vi "SMU Switch Handshaking - 1A - 2810 - Ba.vi"(8 "error in":errorcluster, 11 "file path (use dialog)":path=path "C:/Users/IES/Desktop/jsontestfile.json") -> (0 "error out":errorcluster, 1 "Ba Results":T1[](array[typedef]) {"Impedance" format="%#_6p"; "Negative Voltage" format="%#_6p"; "Positive Voltage" format="%#_6p"}, 2 "Results":T4={"R ch0 Array"=[2.6402355104591723e-06, 3.2050422226470716e-06, 3.2738385547093894e-06, 3.0004056082675545e-06, 3.190429018678622e-06, 3.265655292871135e-06, 3.4283206777974678e-06], "R ch1 Array"=[3.579181433209794e-06, 3.538102305000126e-06, 3.3674070559982216e-06, 3.2951997357567907e-06, 3.0614196043446336e-06, 3.247982674682344e-06, 3.4582756481500834e-06], "R ch2 Array"=[2.636942617106564e-06, 2.444215695573972e-06, 2.3600385872845126e-06, 2.3785120159418297e-06, 2.39158079459529e-06, 2.5415574149365358e-06, 2.629696833600491e-06], "R ch3 Array"=[4.29015971742814e-06, 4.582682915243894e-06, 4.199947801068903e-06, 4.210565880465411e-06, 4.1249236933492e-06, 4.3283146693326225e-06], "R ch4 Array"=[3.2068632920738282e-06, 3.2352868353418705e-06, 3.218523090660476e-06, 3.1985005992771743e-06, 3.2252632419667723e-06, 3.3472279144313767e-06], "R ch5 Array"=[4.190513905088153e-06, 4.23972086032935e-06, 4.053579560688339e-06, 3.9410571545407844e-06, 4.234836387112458e-06, 4.06030163753006e-06], "Elapsed Time (ms)"=11164, "SMU Fault Array"=[], "DMM Fault Array"=[]} {"R ch0 Array" format="%#_6p"; "R ch3 Array" format="%#_6p"; "R ch1 Array" format="%#_6p"; "R ch4 Array" format="%#_6p"; "R ch2 Array" format="%#_6p"; "R ch5 Array" format="%#_6p"}, 3 "Elapsed Time":u32)   [LabVIEW 2019]
uses:
  Results.ctl
  <instrlib>/niDMM/nidmm.llb/niDMM Acquisition State.ctl
  Labview-grpc-measurement-server-master/VIs/MeasurementServer_FourProbeRawData.ctl
  Labview-grpc-measurement-server-master/VIs/MeasurementServer_ErrorOutData.ctl
  JSONCluster.ctl
  <instrlib>/niDCPower/nidcpower.llb/niDCPower Send Software Edge Trigger - Signal.ctl
  <instrlib>/niSwitch/niSwitch.llb/niSwitch Topologies.ctl
  <instrlib>/niDMM/nidmm.llb/niDMM Configure Measurement Absolute.vi
  <instrlib>/niDCPower/nidcpower.llb/niDCPower Configure Software Edge Start Trigger.vi
  <instrlib>/niDCPower/nidcpower.llb/niDCPower Configure Software Edge Sequence Advance Trigger.vi
  <instrlib>/niSwitch/niSwitch.llb/niSwitch Connect Channels (Multiple).vi
  <instrlib>/niSwitch/niSwitch.llb/niSwitch Connect Channels (Single).vi
  <instrlib>/niSwitch/niSwitch.llb/niSwitch Disconnect Channels (Single).vi
  <instrlib>/niSwitch/niSwitch.llb/niSwitch Disconnect Channels (Multiple).vi
  Labview-grpc-measurement-server-master/VIs/labview-grpc-measurement-server.lvlib
panel:
  out "Acq State":T3 caption="Acquisition State"
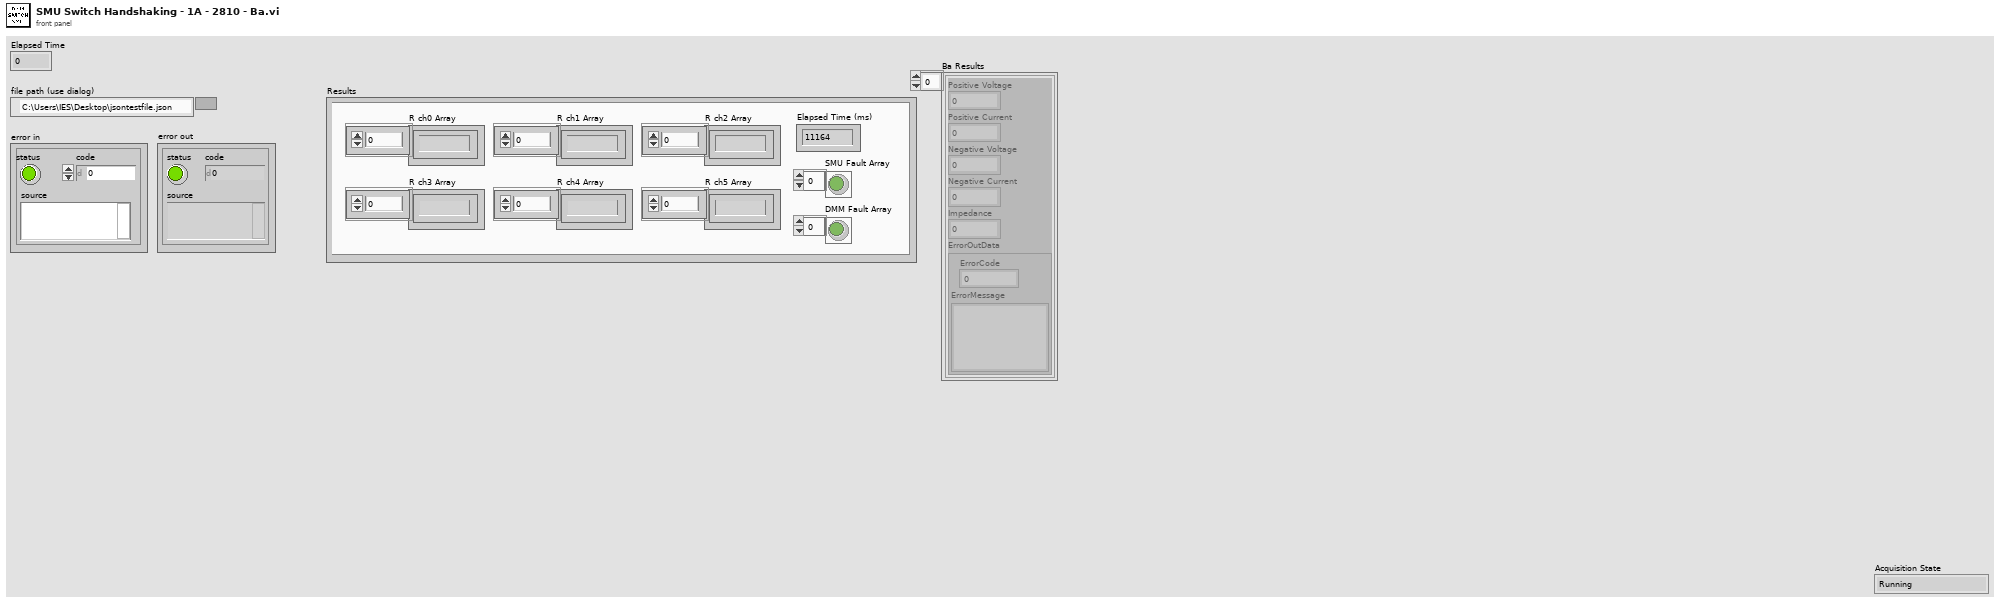
[diagram p1: front panel]
types:
  T1 = typedef "labview-grpc-measurement-server.lvlib/MeasurementServer_FourProbeRawData.ctl" = cluster{"Positive Voltage":sgl, "Positive Current":sgl, "Negative Voltage":sgl, "Negative Current":sgl, "Impedance":sgl, "ErrorOutData":T2}
  T2 = typedef "labview-grpc-measurement-server.lvlib/MeasurementServer_ErrorOutData.ctl" = cluster{"ErrorCode":i32, "ErrorMessage":string}
  T3 = typedef "niDMM Acquisition State.ctl" = enum16{"Running", "Finished with Backlog", "Finished with no Backlog", "Paused", "No acquisition in progress"}
  T4 = typedef "Results.ctl" = cluster{"R ch0 Array":dbl[], "R ch1 Array":dbl[], "R ch2 Array":dbl[], "R ch3 Array":dbl[], "R ch4 Array":dbl[], "R ch5 Array":dbl[], "Elapsed Time (ms)":u32, "SMU Fault Array":bool[], "DMM Fault Array":bool[]}
  T5 = typedef "niSwitch Topologies.ctl" = string
  T6 = typedef "niDCPower Send Software Edge Trigger - Signal.ctl" = i32
  T7 = typedef "JSONCluster.ctl" = cluster{"SMUResourceName":string, "SMUChannels":string, "SMUSourceMode_Sequence":i32, "SMUOutputFunction_DCCurrent":i32, "SMUSourceTransientResponse_Fast":i32, "SMUCurrent":dbl, "SMUCurrentLevelRange":dbl, "SMUMeasurementSense_Local":i32, "SMUMeasurementApertureTime":dbl, "SMUSourceAdvancedSourceDelay":dbl, "SMUVoltage":dbl, "SMUSourceAdvancedSequenceLoopCount":i32, "SMUMeasurementAdvancedDCNoiseRejection_Normal":i32, "SMUSequenceName":string, "SMUStep1_Source_DCCurrent_CurrentLevel":i32, "SMUStep2_Measurement_ApertureTime":i32, "SMUStep3_Source_Advanced_SourceDelay":i32, "SMUSequenceNumberOfSteps":i32, "SMUTriggerFromSwitch_StartDigitalEdge":string, "SMUTriggerFromSwitch_SequenceAdvanceDigitalEdge":string, "SMUTriggerToDMM_SourceCompleteEvent":i32, "SMUTriggerToDMM_SourceCompleteEvent_Value":string, "SMUTriggerToSwitch_SequenceIterationCompleteEvent":i32, "SMUTriggerToDMM_SequenceIterationCompleteEvent_Value":string, "SwitchResourceName":string, "SwitchTopology":string, "SwitchInputTrigger_TTL0":i32, "SwitchScanAdvancedOutput_TTL1":i32, "SwitchScanList":string, "DMMResourceName":string, "DMMFunction_DCVolts":i32, "DMMResolution":dbl, "DMMRange":dbl, "DMMTriggerSource_TTL2":i32, "DMMTriggerSlope_RisingEdge":i32, "DMMSampleTrigger_TTL2":i32, "DMMSampleCount":i32, "DMMSampleTriggerSlope_RisingEdge":i32, "DMMApertureTimeUnits_Seconds":i32, "DMMApertureTime":dbl, "DMMNumberOfAverages":i32, "DMMAutoZero_Off":i32, "DMMADCCalibration_Off":i32, "DMMSettleTime":dbl, "DMMControlAction_Commit":i32, "ApplicationNumberOfWeldChannels":i32}
  T8 = enum16{"open", "replace", "create", "open or create", "replace or create", "replace or create with confirmation"}
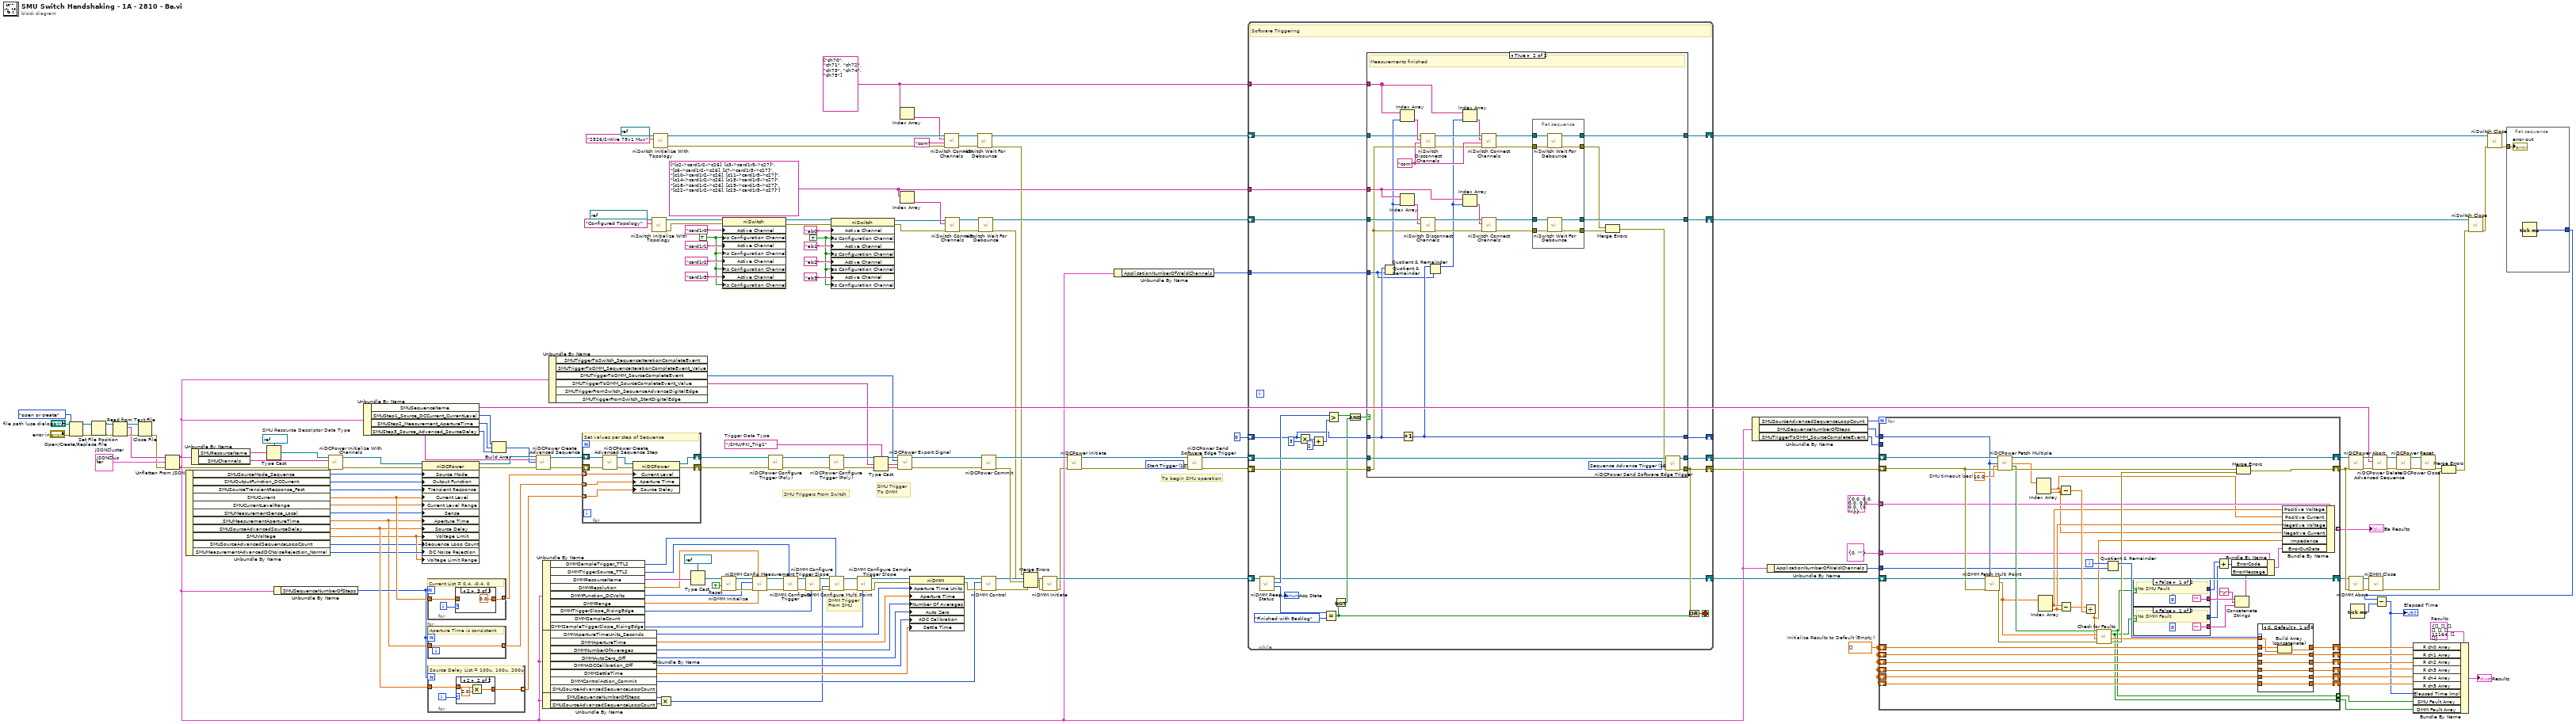
[diagram p0: block diagram]
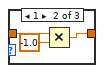
[diagram p4: hidden frame]
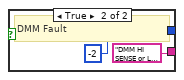
[diagram p6: hidden frame]
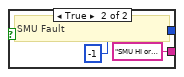
[diagram p7: hidden frame]
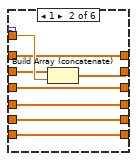
[diagram p8: hidden frame]
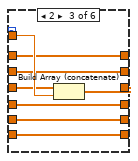
[diagram p9: hidden frame]
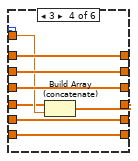
[diagram p10: hidden frame]
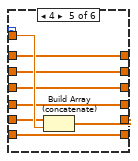
[diagram p11: hidden frame]
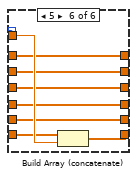
[diagram p12: hidden frame]
diagram:
  w10 = string[] ["ch70", "ch71", "ch72", "ch73", "ch74", "ch75"] ("2525 Scan List Channels")
  w22 = TRUE ("Channel Configuration:Analog Bus Sharing Enable")
  w35 = string[] ["[c2->card1r2->c26], [c3->card1r3->c27]", "[c6->card1r2->c26], [c7->card1r3->c27]", "[c10->card1r2->c26], [c11->card1r3->c27]", "[c14->card1r2->c26], [c15->card1r3->c27]", "[c18->card1r2->c26], [c19->card1r3->c27]", "[c22->card1r2->c26], [c23->card1r3->c27]"]
  w36 = TRUE ("Channel Configuration:Is Source Channel")
  w57 = T6 1034 items=["Start Trigger"=1034, "Source Trigger"=1035, "Measure Trigger"=1036, "Sequence Advance Trigger"=1037, "Pulse Trigger"=1053] ("signal")
  w134 = refnum<k15> "SMU"  # SMU Resource Descriptor Data Type
  w130 = T7 {"SMUResourceName"="", "SMUChannels"="", "SMUSourceMode_Sequence"=0, "SMUOutputFunction_DCCurrent"=0, "SMUSourceTransientResponse_Fast"=0, "SMUCurrent"=0.0, "SMUCurrentLevelRange"=0.0, "SMUMeasurementSense_Local"=0, "SMUMeasurementApertureTime"=0.0, "SMUSourceAdvancedSourceDelay"=0.0, "SMUVoltage"=0.0, "SMUSourceAdvancedSequenceLoopCount"=0, "SMUMeasurementAdvancedDCNoiseRejection_Normal"=0, "SMUSequenceName"="", "SMUStep1_Source_DCCurrent_CurrentLevel"=0, "SMUStep2_Measurement_ApertureTime"=0, "SMUStep3_Source_Advanced_SourceDelay"=0, "SMUSequenceNumberOfSteps"=0, "SMUTriggerFromSwitch_StartDigitalEdge"="", "SMUTriggerFromSwitch_SequenceAdvanceDigitalEdge"="", "SMUTriggerToDMM_SourceCompleteEvent"=0, "SMUTriggerToDMM_SourceCompleteEvent_Value"="", "SMUTriggerToSwitch_SequenceIterationCompleteEvent"=0, "SMUTriggerToDMM_SequenceIterationCompleteEvent_Value"="", "SwitchResourceName"="", "SwitchTopology"="", "SwitchInputTrigger_TTL0"=0, "SwitchScanAdvancedOutput_TTL1"=0, "SwitchScanList"="", "DMMResourceName"="", "DMMFunction_DCVolts"=0, "DMMResolution"=0.0, "DMMRange"=0.0, "DMMTriggerSource_TTL2"=0, "DMMTriggerSlope_RisingEdge"=0, "DMMSampleTrigger_TTL2"=0, "DMMSampleCount"=0, "DMMSampleTriggerSlope_RisingEdge"=0, "DMMApertureTimeUnits_Seconds"=0, "DMMApertureTime"=0.0, "DMMNumberOfAverages"=0, "DMMAutoZero_Off"=0, "DMMADCCalibration_Off"=0, "DMMSettleTime"=0.0, "DMMControlAction_Commit"=0, "ApplicationNumberOfWeldChannels"=0}  # JSONCluster
  w115 = T4 {"R ch0 Array"=[], "R ch1 Array"=[], "R ch2 Array"=[], "R ch3 Array"=[], "R ch4 Array"=[], "R ch5 Array"=[], "Elapsed Time (ms)"=11164, "SMU Fault Array"=[], "DMM Fault Array"=[]}  # Results
  w117 = dbl[] []  # Initialize Results to Default (Empty)
  w162 = TRUE  # Reset
  w84 = tag "/SMU/PXI_Trig1"  # Trigger Data Type
  # "To begin SMU operation"
  # "DMM Trigger\nFrom SMU"
  # "SMU Trigger \nTo DMM"
  # "SMU Triggers From Switch"
  n1 = Open/Create/Replace File(file path (use dialog)="file path (use dialog)", error in="error in", operation (0:open)=T8."open or create") -> (refnum out=w123:refnum<file>, error out=w122:errorcluster)  [unwired: 3 in, 1 out]
  n2 = Set File Position(refnum=w123, error in=w122) -> (refnum out=w125:refnum<file>, error out=w124:errorcluster)  [unwired: 2 in]
  n3 = Read from Text File(file (use dialog)=w125, error in=w124) -> (refnum out=w127:refnum<file>, text=w121:string, error out=w126:errorcluster)  [unwired: 2 in, 1 out]
  n4 = Close File(refnum=w127, error in=w126) -> (error out=w120:errorcluster)  [unwired: 1 out]
  n5 = Unflatten From JSON(JSON string=w121, type and defaults=w130, error in (no error)=w120) -> (value=w47:T7, error out=w119:errorcluster)  [unwired: 4 in]
  n6 = Unbundle By Name(w47) -> ("SMUSourceMode_Sequence"=w97:i32, "SMUOutputFunction_DCCurrent"=w96:i32, "SMUSourceTransientResponse_Fast"=w102:i32, "SMUCurrent"=w101:dbl, "SMUCurrentLevelRange"=w100:dbl, "SMUMeasurementSense_Local"=w99:i32, "SMUMeasurementApertureTime"=w6:dbl, "SMUSourceAdvancedSourceDelay"=w98:dbl, "SMUVoltage"=w94:dbl, "SMUSourceAdvancedSequenceLoopCount"=w69:i32, "SMUMeasurementAdvancedDCNoiseRejection_Normal"=w95:i32)
  n7 = Unbundle By Name(w47) -> ("SMUResourceName"=w132:string, "SMUChannels"=w131:string)
  n8 = Type Cast(type=w134, x=w132) -> (*(type *) &x=w133:refnum<k15>)
  n9 = Unbundle By Name(w47) -> ("SMUSequenceNumberOfSteps"=w92:i32)
  n10 = call <instrlib>:"niDCPower Initialize With Channels.vi"("error in (no error)"=w119, "channels"=w131, "resource name"=w133) -> ("error out"=w181:errorcluster, "instrument handle out"=w182:refnum<k15>)  [unwired: 7 in]
  n11 = Unbundle By Name(w47) -> ("SMUSequenceName"=w88:string, "SMUStep1_Source_DCCurrent_CurrentLevel"=w91:i32, "SMUStep2_Measurement_ApertureTime"=w90:i32, "SMUStep3_Source_Advanced_SourceDelay"=w89:i32)
  n12 = property class="niDCPower"(reference=w182, error in=w181, "Source Mode"=w97, "Output Function"=w96, "Transient Response"=w102, "Current Level"=w101, "Current Level Range"=w100, "Sense"=w99, "Aperture Time"=w6, "Source Delay"=w98, "Voltage Limit"=w94, "Sequence Loop Count"=w69, "DC Noise Rejection"=w95, "Voltage Limit Range"=w94) -> (reference out=w176:refnum<k15>, error out=w175:errorcluster)
  n13 = for {
    N: w92 -> [_]
    tunnel: w101 -> [w184]
    tunnel: [w183] -> w105 mode=indexing
    i -> [w185]
    # "Current List = 0.4, -0.4, 0"
    n14 = case shown="2" w185 {
      tunnel: w184 -> [w186 w188 _]
      tunnel: [w186 w189 0.0 ("current")] -> w183
      frame 0, Default {
      }
      frame 1 {
        n15 = Multiply(x=w188, y=-1.0) -> (x*y=w189:dbl)
      }
      frame 2 {
      }
    }
  }
  n16 = for {
    N: w92 -> [_]
    tunnel: w6 -> [w191]
    tunnel: [w191] -> w104 mode=indexing
    # "Aperture Time is consistent"
  }
  n17 = for {
    N: w92 -> [_]
    tunnel: w98 -> [w194]
    tunnel: [w193] -> w103 mode=indexing
    i -> [w192]
    # "Source Delay List = 100u, 100u, 200u"
    n18 = case shown="2" w192 {
      tunnel: w194 -> [w195 w198]
      tunnel: [w195 w196] -> w193
      frame 0, Default {
      }
      frame 2 {
        n19 = Multiply(x=w198, y=2.0) -> (x*y=w196:dbl)
      }
    }
  }
  n20 = Build Array(w91, w90, w89) -> (w93:i32[])
  n21 = call <instrlib>:"niDCPower Create Advanced Sequence.vi"("instrument handle"=w176, "sequence name"=w88, "advanced sequence properties"=w93, "error in (no error)"=w175) -> ("instrument handle out"=w168:refnum<k15>, "error out"=w167:errorcluster)  [unwired: 10 in]
  n22 = Unbundle By Name(w47) -> ("DMMSampleTrigger_TTL2"=w76:i32, "DMMTriggerSource_TTL2"=w81:i32, "DMMResourceName"=w64:string, "DMMResolution"=w63:dbl, "DMMFunction_DCVolts"=w78:i32, "DMMRange"=w80:dbl, "DMMTriggerSlope_RisingEdge"=w79:i32, "DMMSampleTriggerSlope_RisingEdge"=w77:i32)  [unwired: 1 out]
  n23 = Unbundle By Name(w47) -> ("DMMApertureTimeUnits_Seconds"=w75:i32, "DMMApertureTime"=w5:dbl, "DMMNumberOfAverages"=w74:i32, "DMMAutoZero_Off"=w73:i32, "DMMADCCalibration_Off"=w72:i32, "DMMSettleTime"=w71:dbl, "DMMControlAction_Commit"=w70:i32)  [unwired: 1 out]
  n24 = Unbundle By Name(w47) -> ("SMUSequenceNumberOfSteps"=w53:i32, "SMUSourceAdvancedSequenceLoopCount"=w52:i32)
  n25 = Unbundle By Name(w47) -> ("SMUTriggerToDMM_SourceCompleteEvent"=w87:i32, "SMUTriggerToDMM_SourceCompleteEvent_Value"=w85:string)  [unwired: 4 out]
  n26 = for {
    shift-right: [w204] -> w165
    shift-left: w167 -> [w207]
    shift-right: [w203] -> w166
    shift-left: w168 -> [w202]
    tunnel: w103 -> [w201] mode=indexing
    tunnel: w105 -> [w199] mode=indexing
    tunnel: w104 -> [w200] mode=indexing
    # "Set values per step of Sequence"
    n27 = call <instrlib>:"niDCPower Create Advanced Sequence Step.vi"("error in (no error)"=w207, "instrument handle"=w202) -> ("error out"=w205:errorcluster, "instrument handle out"=w206:refnum<k15>)  [unwired: 8 in]
    n28 = property class="niDCPower"(reference=w206, error in=w205, "Current Level"=w199, "Aperture Time"=w200, "Source Delay"=w201) -> (reference out=w203:refnum<k15>, error out=w204:errorcluster)
  }
  n29 = call <instrlib>:"niSwitch Initialize With Topology.vi"("topology name"=T5 "Configured Topology", "resource name"=refnum<k15> "SwitchBlock1Dev1") -> ("error out"=w41:errorcluster, "instrument handle out"=w42:refnum<k15>)  [unwired: 3 in, 5 out]
  n30 = call <instrlib>:"niSwitch Initialize With Topology.vi"("topology name"=T5 "2526/2-Wire 79x1 Mux", "resource name"=refnum<k15> "2526_1") -> ("error out"=w18:errorcluster, "instrument handle out"=w19:refnum<k15>)  [unwired: 3 in, 5 out]
  n31 = Multiply(x=w53, y=w52) -> (x*y=w51:i32)
  n32 = Type Cast(type=refnum<k15> "DMM" ("Device Name"), x=w64) -> (*(type *) &x=w82:refnum<k15>)
  n33 = call <instrlib>:"niDMM Initialize.vi"("Reset"=w162, "Instrument Descriptor"=w82) -> ("error out"=w151:errorcluster, "instrument handle out"=w150:refnum<k15>)  [unwired: 8 in]
  n34 = property class="niSwitch"(reference=w42, error in=w41, "Active Channel"="card1r0", "Is Configuration Channel"=w36, "Active Channel"="card1r1", "Is Configuration Channel"=w36, "Active Channel"="card1r2", "Is Configuration Channel"=w36, "Active Channel"="card1r3", "Is Configuration Channel"=w36) -> (reference out=w30:refnum<k15>, error out=w29:errorcluster)
  n35 = call-poly <instrlib>:"niDMM Config Measurement.vi"("Range"=w80, "Resolution"=w63, "error in (no error)"=w151, "Function"=w78, "instrument handle"=w150) -> ("error out"=w155:errorcluster, "instrument handle out"=w154:refnum<k15>)  [unwired: 5 in]
  n36 = call-poly <instrlib>:"niDCPower Configure Trigger (Poly).vi"("error in (no error)"=w165, "instrument handle"=w166) -> ("error out"=w178:errorcluster, "instrument handle out"=w179:refnum<k15>)  [unwired: 8 in]
  n37 = call <instrlib>:"niDMM Configure Trigger.vi"("Trigger Source"=w81, "error in (no error)"=w155, "instrument handle"=w154) -> ("error out"=w157:errorcluster, "instrument handle out"=w156:refnum<k15>)  [unwired: 7 in]
  n38 = call <instrlib>:"niDMM Configure Trigger Slope.vi"("Slope"=w79, "error in (no error)"=w157, "instrument handle"=w156) -> ("error out"=w159:errorcluster, "instrument handle out"=w158:refnum<k15>)  [unwired: 7 in]
  n39 = call-poly <instrlib>:"niDCPower Configure Trigger (Poly).vi"("error in (no error)"=w178, "instrument handle"=w179) -> ("error out"=w135:errorcluster, "instrument handle out"=w136:refnum<k15>)  [unwired: 8 in]
  n40 = call <instrlib>:"niDMM Configure Multi Point.vi"("Sample Trigger"=w76, "error in (no error)"=w159, "Sample Count"=w51, "instrument handle"=w158) -> ("error out"=w161:errorcluster, "instrument handle out"=w160:refnum<k15>)  [unwired: 6 in]
  n41 = property class="niSwitch"(reference=w30, error in=w29, "Active Channel"="ab0", "Is Configuration Channel"=w22, "Active Channel"="ab1", "Is Configuration Channel"=w22, "Active Channel"="ab2", "Is Configuration Channel"=w22, "Active Channel"="ab3", "Is Configuration Channel"=w22) -> (reference out=w28:refnum<k15>, error out=w27:errorcluster)
  n42 = call <instrlib>:"niDMM Configure Sample Trigger Slope.vi"("Slope"=w77, "error in (no error)"=w161, "instrument handle"=w160) -> ("error out"=w143:errorcluster, "instrument handle out"=w144:refnum<k15>)  [unwired: 7 in]
  n43 = Type Cast(type=w84, x=w85) -> (*(type *) &x=w86:tag)
  n44 = call <instrlib>:"niDCPower Export Signal.vi"("error in (no error)"=w135, "output terminal"=w86, "signal"=w87, "instrument handle"=w136) -> ("error out"=w163:errorcluster, "instrument handle out"=w164:refnum<k15>)  [unwired: 6 in]
  n45 = Index Array(array=w10) -> (element=w17:string)  [unwired: 1 in]
  n46 = Index Array(array=w35) -> (element=w48:string)  [unwired: 1 in]
  n47 = property class="niDMM"(reference=w144, error in=w143, "Aperture Time Units"=w75, "Aperture Time"=w5, "Number Of Averages"=w74, "Auto Zero"=w73, "ADC Calibration"=w72, "Settle Time"=w71) -> (reference out=w138:refnum<k15>, error out=w137:errorcluster)
  n48 = call-poly <instrlib>:"niSwitch Connect Channels.vi"("error in (no error)"=w18, "channel 2"="com", "channel 1"=w17, "instrument handle"=w19) -> ("error out"=w14:errorcluster, "instrument handle out"=w15:refnum<k15>)  [unwired: 6 in]
  n49 = call-poly <instrlib>:"niSwitch Connect Channels.vi"("error in (no error)"=w27, "connection list"=w48, "instrument handle"=w28) -> ("error out"=w33:errorcluster, "instrument handle out"=w34:refnum<k15>)  [unwired: 7 in]
  n50 = call <instrlib>:"niSwitch Wait For Debounce.vi"("error in (no error)"=w14, "instrument handle"=w15) -> ("error out"=w12:errorcluster, "instrument handle out"=w11:refnum<k15>)  [unwired: 8 in]
  n51 = call <instrlib>:"niSwitch Wait For Debounce.vi"("error in (no error)"=w33, "instrument handle"=w34) -> ("error out"=w32:errorcluster, "instrument handle out"=w31:refnum<k15>)  [unwired: 8 in]
  n52 = call <instrlib>:"niDCPower Commit.vi"("error in (no error)"=w163, "instrument handle"=w164) -> ("error out"=w149:errorcluster, "instrument handle out"=w146:refnum<k15>)  [unwired: 8 in]
  n53 = call <instrlib>:"niDMM Control.vi"("error in (no error)"=w137, "Control Action"=w70, "instrument handle"=w138) -> ("error out"=w148:errorcluster, "instrument handle out"=w145:refnum<k15>)  [unwired: 7 in]
  n54 = Merge Errors(w12, w32, w149, w148) -> (w147:errorcluster)
  n55 = call <instrlib>:"niDMM Initiate.vi"("error in (no error)"=w147, "instrument handle"=w145) -> ("error out"=w13:errorcluster, "instrument handle out"=w56:refnum<k15>)  [unwired: 8 in]
  n56 = call <instrlib>:"niDCPower Initiate.vi"("error in (no error)"=w13, "instrument handle"=w146) -> ("error out"=w45:errorcluster, "instrument handle out"=w60:refnum<k15>)  [unwired: 8 in]
  n57 = Unbundle By Name(w47) -> ("ApplicationNumberOfWeldChannels"=w46:i32)
  n58 = call <instrlib>:"niDCPower Send Software Edge Trigger.vi"("error in (no error)"=w45, "signal"=w57, "instrument handle"=w60) -> ("error out"=w58:errorcluster, "instrument handle out"=w59:refnum<k15>)  [unwired: 7 in]
  n59 = while {
    shift-right: [w234] -> w62
    shift-left: w59 -> [w229]
    shift-right: [w232] -> w61
    shift-left: w58 -> [w228]
    shift-right: [w230] -> w49
    shift-left: w31 -> [w231]
    shift-right: [w223] -> w55
    shift-left: w56 -> [w224]
    shift-right: [w217] -> _
    shift-left: 0 ("Backlog") -> [w218]
    tunnel: w35 -> [w212]
    tunnel: w46 -> [w211]
    shift-right: [w209] -> w9
    shift-left: w11 -> [w210]
    tunnel: w10 -> [w208]
    stop <- w233 stop-if-true
    # "Software Triggering"
    n60 = call <instrlib>:"niDMM Read Status.vi"("instrument handle"=w224) -> ("Acquisition State"=w227:T3, "Backlog"=w225:i32, "instrument handle out"=w223:refnum<k15>)  [unwired: 7 in, 1 out]
    "Acq State" <- w227
    n61 = Multiply(x=w218, y=3) -> (x*y=w220:i32)
    n62 = Add(x=w220, y=2) -> (x+y=w221:i32)
    n63 = Equal?(x=w227, y=niDMM_Acquisition_State."Finished with Backlog") -> (x = y?=w216:bool)
    n64 = Greater?(x=w225, y=w221) -> (0:w215:bool)
    n65 = Not(x=w216) -> (.not. x?=w214:bool)
    n66 = And(x=w215, y=w214) -> (x .and. y?=w213:bool)
    n67 = case shown="True" w213 {
      tunnel: w228 -> [w238 w243]
      tunnel: [w239 w271] -> w234
      tunnel: [w238 w270] -> w232
      tunnel: w229 -> [w239 w267]
      tunnel: w231 -> [w237 w266]
      tunnel: [w237 w269] -> w230
      tunnel: w218 -> [w236 w259]
      tunnel: [w236 w258] -> w217
      tunnel: w212 -> [_ w262]
      tunnel: w211 -> [_ w257]
      tunnel: w210 -> [w235 w248]
      tunnel: [w235 w245] -> w209
      tunnel: w208 -> [_ w244]
      frame False {
        # "Measurements not finished yet - repeat loop"
      }
      frame True {
        w252 = "com" ("channel 2")
        w268 = T6 1037 items=["Start Trigger"=1034, "Source Trigger"=1035, "Measure Trigger"=1036, "Sequence Advance Trigger"=1037, "Pulse Trigger"=1053] ("signal")
        # "Measurements finished"
        n68 = Quotient & Remainder(x=w259, y=w257) -> (x-y*floor(x/y)=w250:i32)  [unwired: 1 out]
        n69 = Index Array(array=w244, index=w250) -> (element=w255:string)
        n70 = Index Array(array=w262, index=w250) -> (element=w265:string)
        n71 = Increment(x=w259) -> (x+1=w258:i32)
        n72 = call-poly <instrlib>:"niSwitch Disconnect Channels.vi"("error in (no error)"=w243, "channel 2"=w252, "channel 1"=w255, "instrument handle"=w248) -> ("error out"=w251:errorcluster, "instrument handle out"=w254:refnum<k15>)  [unwired: 6 in]
        n73 = call-poly <instrlib>:"niSwitch Disconnect Channels.vi"("error in (no error)"=w243, "disconnection list"=w265, "instrument handle"=w266) -> ("error out"=w260:errorcluster, "instrument handle out"=w264:refnum<k15>)  [unwired: 7 in]
        n74 = Quotient & Remainder(x=w258, y=w257) -> (x-y*floor(x/y)=w249:i32)  [unwired: 1 out]
        n75 = Index Array(array=w244, index=w249) -> (element=w253:string)
        n76 = Index Array(array=w262, index=w249) -> (element=w261:string)
        n77 = call-poly <instrlib>:"niSwitch Connect Channels.vi"("error in (no error)"=w251, "channel 2"=w252, "channel 1"=w253, "instrument handle"=w254) -> ("error out"=w246:errorcluster, "instrument handle out"=w247:refnum<k15>)  [unwired: 6 in]
        n78 = call-poly <instrlib>:"niSwitch Connect Channels.vi"("error in (no error)"=w260, "connection list"=w261, "instrument handle"=w264) -> ("error out"=w256:errorcluster, "instrument handle out"=w263:refnum<k15>)  [unwired: 7 in]
        n79 = flat-sequence {
          tunnel: [w279] -> w269
          tunnel: [w278] -> w242
          tunnel: w263 -> [w277]
          tunnel: w256 -> [w276]
          tunnel: w247 -> [w275]
          tunnel: w246 -> [w274]
          tunnel: [w273] -> w245
          tunnel: [w272] -> w241
          frame #0 {
            n80 = call <instrlib>:"niSwitch Wait For Debounce.vi"("error in (no error)"=w274, "instrument handle"=w275) -> ("error out"=w272:errorcluster, "instrument handle out"=w273:refnum<k15>)  [unwired: 8 in]
            n81 = call <instrlib>:"niSwitch Wait For Debounce.vi"("error in (no error)"=w276, "instrument handle"=w277) -> ("error out"=w278:errorcluster, "instrument handle out"=w279:refnum<k15>)  [unwired: 8 in]
          }
        }
        n82 = Merge Errors(w241, w242) -> (w240:errorcluster)
        n83 = call <instrlib>:"niDCPower Send Software Edge Trigger.vi"("error in (no error)"=w240, "signal"=w268, "instrument handle"=w267) -> ("error out"=w270:errorcluster, "instrument handle out"=w271:refnum<k15>)  [unwired: 7 in]
      }
    }
    n84 = Or(x=w232, y=w216) -> (x .or. y?=w233:bool)
  }
  n85 = Unbundle By Name(w47) -> ("SMUSourceAdvancedSequenceLoopCount"=w68:i32, "SMUSequenceNumberOfSteps"=w67:i32, "SMUTriggerToDMM_SourceCompleteEvent"=w66:i32)
  n86 = Unbundle By Name(w47) -> ("ApplicationNumberOfWeldChannels"=w65:i32)
  n87 = for {
    N: w68 -> [_]
    tunnel: w67 -> [w302]
    shift-right: [w324] -> w142
    shift-left: w61 -> [w303]
    shift-right: [w329] -> w180
    shift-left: w62 -> [w304]
    shift-right: [w292] -> w139
    shift-left: w55 -> [w326]
    shift-right: [w323] -> w116
    shift-left: w117 -> [w322]
    shift-right: [w321] -> w110
    shift-left: w117 -> [w320]
    shift-right: [w319] -> w111
    shift-left: w117 -> [w318]
    shift-right: [w317] -> w112
    shift-left: w117 -> [w316]
    shift-right: [w315] -> w113
    shift-left: w117 -> [w314]
    shift-right: [w313] -> w114
    shift-left: w117 -> [w312]
    tunnel: [w287] -> w107 mode=indexing
    tunnel: [w283] -> w106 mode=indexing
    tunnel: w66 -> [_]
    tunnel: w65 -> [w301]
    tunnel: T1 {"Positive Voltage"=0.0, "Positive Current"=0.0, "Negative Voltage"=0.0, "Negative Current"=0.0, "Impedance"=0.0, "ErrorOutData"={"ErrorCode"=0, "ErrorMessage"=""}} ("FourProbeRawData") -> [w298]
    tunnel: T2 {"ErrorCode"=0, "ErrorMessage"=""} ("ErrorOutData") -> [w290]
    tunnel: [w289] -> w2 mode=indexing
    i -> [w328]
    w307 = 10.0  # SMU timeout (sec)
    n88 = call <instrlib>:"niDMM Fetch Multi Point.vi"("Number to Fetch"=w302, "error in (no error)"=w303, "instrument handle"=w326) -> ("error out"=w310:errorcluster, "Measurements"=w299:dbl[], "instrument handle out"=w292:refnum<k15>)  [unwired: 5 in, 1 out]
    n89 = call <instrlib>:"niDCPower Fetch Multiple.vi"("instrument handle"=w304, "count (1)"=w302, "timeout (sec)"=w307, "error in (no error)"=w303) -> ("instrument handle out"=w329:refnum<k15>, "current measurements"=w300:dbl[], "in compliance"=w311:bool[], "error out"=w325:errorcluster)  [unwired: 6 in, 2 out]
    n90 = Index Array(array=w300) -> (element #1=w296:dbl, element #2=w294:dbl)  [unwired: 2 in]
    n91 = Index Array(array=w299) -> (element #1=w297:dbl, element #2=w295:dbl)  [unwired: 2 in]
    n92 = Subtract(x=w296, y=w294) -> (x-y=w306:dbl)
    n93 = Subtract(x=w297, y=w295) -> (x-y=w305:dbl)
    n94 = Divide(x=w305, y=w306) -> (x/y=w293:dbl)
    n95 = call "Check for Faults.vi"("Error In"=w310, "Resistance In"=w293, "dmm voltage measurements"=w299, "in compliance"=w311) -> ("Error Out"=w309:errorcluster, "Resistance Out"=w308:dbl, "DMM Fault"=w283:bool, "SMU Fault"=w287:bool)  [unwired: 4 in]
    n96 = Quotient & Remainder(x=w328, y=w301) -> (x-y*floor(x/y)=w327:i32)  [unwired: 1 out]
    n97 = case shown="False" w287 {
      tunnel: ["" "SMU HI or LO lead disconnected\n- SMU in compliance\n- SMU Fault = True"] -> w286
      tunnel: [0 -1] -> w284
      frame False {
        # "No SMU Fault"
      }
      frame True {
        # "SMU Fault"
      }
    }
    n98 = case shown="False" w283 {
      tunnel: ["" "DMM HI SENSE or LO SENSE lead disconnected\n- DMM measures NaN, or \n- DMM overrange warning, or\n- DMM voltage > 50uV "] -> w281
      tunnel: [0 -2] -> w280
      frame False {
        # "No DMM Fault"
      }
      frame True {
        # "DMM Fault"
      }
    }
    n99 = Add(x=w284, y=w280) -> (x+y=w288:i32)
    n100 = Concatenate Strings(w286, "\r", w281) -> (w285:string)
    n101 = Bundle By Name(cluster=w290, "ErrorCode"=w288, "ErrorMessage"=w285) -> (w291:T2)
    n102 = Merge Errors(w325, w309) -> (w324:errorcluster)
    n103 = case shown="0, Default" w327 {
      tunnel: w308 -> [w345 w353 w361 w366 w377 w385]
      tunnel: [w344 w350 w358 w369 w374 w382] -> w323
      tunnel: w322 -> [w343 w350 w358 w369 w374 w382]
      tunnel: [w342 w352 w357 w368 w373 w381] -> w321
      tunnel: w320 -> [w342 w351 w357 w368 w373 w381]
      tunnel: [w341 w349 w360 w367 w372 w380] -> w319
      tunnel: w318 -> [w341 w349 w359 w367 w372 w380]
      tunnel: [w340 w348 w356 w365 w371 w379] -> w317
      tunnel: w316 -> [w340 w348 w356 w364 w371 w379]
      tunnel: [w339 w347 w355 w363 w376 w378] -> w315
      tunnel: w314 -> [w339 w347 w355 w363 w375 w378]
      tunnel: [w338 w346 w354 w362 w370 w384] -> w313
      tunnel: w312 -> [w338 w346 w354 w362 w370 w383]
      frame 0, Default {
        n104 = Build Array (concatenate)(w343, w345) -> (w344:dbl[])
      }
      frame 1 {
        n105 = Build Array (concatenate)(w351, w353) -> (w352:dbl[])
      }
      frame 2 {
        n106 = Build Array (concatenate)(w359, w361) -> (w360:dbl[])
      }
      frame 3 {
        n107 = Build Array (concatenate)(w364, w366) -> (w365:dbl[])
      }
      frame 4 {
        n108 = Build Array (concatenate)(w375, w377) -> (w376:dbl[])
      }
      frame 5 {
        n109 = Build Array (concatenate)(w383, w385) -> (w384:dbl[])
      }
    }
    n110 = Bundle By Name(cluster=w298, "Positive Voltage"=w297, "Positive Current"=w296, "Negative Voltage"=w295, "Negative Current"=w294, "Impedance"=w293, "ErrorOutData"=w291) -> (w289:T1)
  }
  "Ba Results" <- w2
  n111 = call <instrlib>:"niDCPower Abort.vi"("error in (no error)"=w142, "instrument handle"=w180) -> ("error out"=w173:errorcluster, "instrument handle out"=w174:refnum<k15>)  [unwired: 8 in]
  n112 = call <instrlib>:"niDMM Abort.vi"("error in (no error)"=w142, "instrument handle"=w139) -> ("error out"=w153:errorcluster, "instrument handle out"=w152:refnum<k15>)  [unwired: 8 in]
  n113 = Tick Count (ms)() -> (millisecond timer value=w177:u32)
  n114 = call <instrlib>:"niDMM Close.vi"("error in (no error)"=w153, "instrument handle"=w152) -> ("error out"=w141:errorcluster)  [unwired: 9 in]
  n115 = call <instrlib>:"niDCPower Delete Advanced Sequence.vi"("error in (no error)"=w173, "sequence name"=w88, "instrument handle"=w174) -> ("error out"=w172:errorcluster, "instrument handle out"=w171:refnum<k15>)  [unwired: 7 in]
  n116 = Subtract(x=w1, y=w177) -> (x-y=w108:u32)
  "Elapsed Time" <- w108
  n117 = call <instrlib>:"niDCPower Reset.vi"("error in (no error)"=w172, "instrument handle"=w171) -> ("error out"=w169:errorcluster, "instrument handle out"=w170:refnum<k15>)  [unwired: 2 in, 6 out]
  n118 = Bundle By Name(cluster=w115, "R ch0 Array"=w116, "R ch1 Array"=w110, "R ch2 Array"=w111, "R ch3 Array"=w112, "R ch4 Array"=w113, "R ch5 Array"=w114, "Elapsed Time (ms)"=w108, "SMU Fault Array"=w107, "DMM Fault Array"=w106) -> (→"Results":T4)
  n119 = call <instrlib>:"niDCPower Close.vi"("error in (no error)"=w169, "instrument handle"=w170) -> ("error out"=w140:errorcluster)  [unwired: 9 in]
  n120 = Merge Errors(w140, w141) -> (w50:errorcluster)
  n121 = call <instrlib>:"niSwitch Close.vi"("error in (no error)"=w50, "instrument handle"=w49) -> ("error out"=w8:errorcluster)  [unwired: 9 out]
  n122 = call <instrlib>:"niSwitch Close.vi"("error in (no error)"=w8, "instrument handle"=w9) -> ("error out"=w7:errorcluster)  [unwired: 9 out]
  n123 = flat-sequence {
    tunnel: w7 -> [w387]
    tunnel: [w386] -> w1
    frame #0 {
      n124 = Tick Count (ms)() -> (millisecond timer value=w386:u32)
      "error out" <- w387
    }
  }
